vi "JoystickStrafeScaling.vi"(3 "Raw Y' Joystick":dbl, 4 "Raw X' Joystick":dbl, 5 "Strafe Deadband":dbl, 6 "Strafe Scaling":dbl) -> (0 "Scaled Y' Joystick":dbl, 1 "Scaled X' Joystick":dbl, 2 "Out of Deadband":bool)   [LabVIEW 2019]
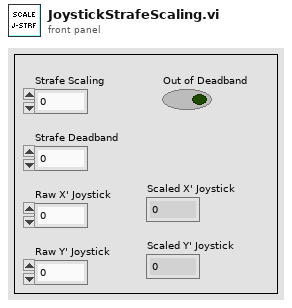
[diagram p1: front panel]
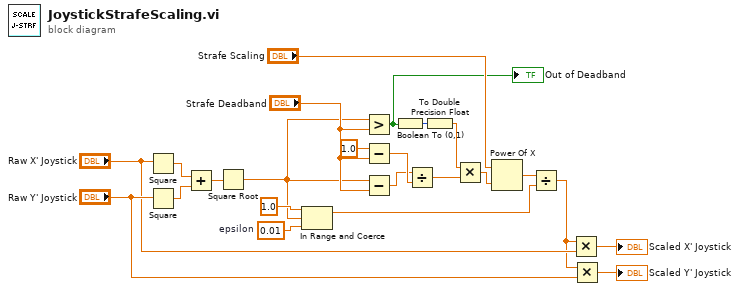
[diagram p0: block diagram]
diagram:
  w11 = 0.01  # epsilon
  n1 = Square(x="Raw X' Joystick") -> (x^2=w8:dbl)
  n2 = Square(x="Raw Y' Joystick") -> (x^2=w7:dbl)
  n3 = Add(x=w8, y=w7) -> (x+y=w9:dbl)
  n4 = Square Root(x=w9) -> (sqrt(x)=w12:dbl)
  n5 = In Range and Coerce(upper limit=1.0, x=w12, lower limit=w11) -> (coerced(x)=w10:dbl)  [unwired: 1 out]
  n6 = Greater?(x=w12, y="Strafe Deadband") -> (0:w19:bool)
  "Out of Deadband" <- w19
  n7 = Subtract(x=1.0, y="Strafe Deadband") -> (x-y=w5:dbl)
  n8 = Subtract(x=w12, y="Strafe Deadband") -> (x-y=w3:dbl)
  n9 = Boolean To (0,1)(Boolean=w19) -> (0, 1=w1:i16)
  n10 = Divide(x=w3, y=w5) -> (x/y=w6:dbl)
  n11 = To Double Precision Float(number=w1) -> (double precision float=w2:dbl)
  n12 = Multiply(x=w2, y=w6) -> (x*y=w21:dbl)
  n13 = Power Of X(1:w21, 2:"Strafe Scaling") -> (0:w22:dbl)
  n14 = Divide(x=w22, y=w10) -> (x/y=w14:dbl)
  n15 = Multiply(x=w14, y="Raw X' Joystick") -> (x*y=→"Scaled X' Joystick":dbl)
  n16 = Multiply(x=w14, y="Raw Y' Joystick") -> (x*y=→"Scaled Y' Joystick":dbl)
